vi "Effective degrees of freedom calculation.vi"(2 "nearest theoretical function from database":dbl[](array[numeric])=[14.666715524342548, 16.90138333280829, 19.565493531663716, 22.468034934420814, 25.369716242622864, 28.014507831534246, 30.16544604921263, 31.639384286174614, 32.33528562740709, 32.25150595291599, 31.48905866982018, 30.23994882008881, 28.76193292452598, 27.343183265376055, 26.26192732565865, 25.746976250071143, 25.94498751581365, 26.899339106940467, 28.543777449264834, 30.71179427774414, 33.160342822507424, 35.604375862397056, 37.75710565967028, 39.370078845854245, 40.26727255385307, 40.36834933783813, 39.69791434607072, 38.37971280154763, 36.61694734948651, 34.66188606250729, 32.77943678304789, 31.21009673576402, 30.137626105997057, 29.6659305163221, 29.80814246726195, 30.489001985309248, 31.55966117680997, 32.82225246541991, 34.06025124495686, 35.06998833065375, 35.68870706219568, 35.815289303031484, 35.42102179832661, 34.54938101853873, 33.30546999892364, 31.837235932372117, 30.311680207906562, 28.889849888622834, 27.704345150070246, 26.842494505993646, 26.337314169172064, 26.167078517448665, 26.262984518631317, 26.523216347810852, 26.830852818485937, 27.072649421221186, 27.155787017237554, 27.020182704278092, 26.644800169957563, 26.04742576452019, 25.27842670219093, 24.409909366263943, 23.522324470978415, 22.690824225874472, 21.973576014511963, 21.403769372456498, 20.986356362346143, 20.699733963447184, 20.50176337963178, 20.338847274488895, 20.156361380280483, 19.908603511423408, 19.566601960763993, 19.122562706598988, 18.5903545705075, 18.00211700795403, 17.40172856792016, 16.83636790594361, 16.347681467955717, 15.964091882344754, 15.695543683815888, 15.531549770559517, 15.442824584109177, 15.386191016951754, 15.311907534335774, 15.172173376651623, 14.929388720572566, 14.562800506093073, 14.072436542779842, 13.47967627959755, 12.82435029809701, 12.158818108287884, 11.539947216562274, 11.020255779363987, 10.639601442195865, 10.418718125431207, 10.355613818743219, 10.425399796133545, 10.583598834475756, 10.772447084026897, 10.929253846443201, 10.9955742344181, 10.925830234343435, 10.694101268139292, 10.298079096445033, 9.759604508936409, 9.121706289664775, 8.442574341744107, 7.787344576171037, 7.218879184426598, 6.788873197068151, 6.53055220457113, 6.453994560675933, 6.544726552242801, 6.765768046685836, 7.062816611730049, 7.37181710788848, 7.62783740408099, 7.77399991658564, 7.769226086789243, 7.593733645058184, 7.251551364867035, 6.7697423925322635, 6.1944854547659425, 5.584594642653517, 5.003403231784681, 4.510140742711135, 4.151991155059185, 3.9578971201764626, 3.93492274116682, 4.0676222706034215, 4.320445857712015, 4.642801727641996, 4.976042598414347, 5.261400575989181, 5.447787979996777, 5.49842305602821, 5.395421935934755, 5.141787446877443, 4.760589240715271, 4.291507174199621, 3.7852569778639444, 3.296687054103397, 2.8774871087765383, 2.569483917826434, 2.3993892663422827, 2.3756550396437954, 2.487793863704487, 2.708190092506199, 2.996098559817216, 3.303249852045647, 3.5802876217834663, 3.783176863206189, 3.878750413061122, 3.8486992279565726, 3.691532066743435, 3.4223110738347264, 3.070261929100643, 2.6746297226566798, 2.2793679210498117], 3 "experimental function":dbl[](array[numeric])=[22.30149557922684, 24.362732109266034, 27.297807376924123, 28.64644784708893, 30.248204511171004, 33.42077097860815, 34.59861401132268, 34.49590803669435, 34.45740788681342, 33.36138072141928, 33.135358407177556, 30.744170387682413, 31.818831427985444, 31.70369415417956, 31.13789549676162, 30.410402938882626, 30.775727742682065, 31.78984571089391, 31.856257108410997, 32.88897866912766, 31.82178580980581, 32.83420528522897, 33.46776374612122, 34.995645227686886, 34.254320967898096, 35.16210631396439, 34.582748836396554, 33.05477293030354, 32.107138663936055, 30.508586238189885, 28.742028842504045, 28.158263200159926, 27.730613373658617, 27.012013000747356, 26.76272642858672, 27.76579503861242, 29.12952017329807, 30.50064773668652, 32.347533632332905, 33.66314575155643, 34.485845630641116, 36.13419599571953, 37.803727241090854, 38.37709300881931, 37.848492410338146, 36.453703555710966, 34.51182843611985, 32.14306663838507, 29.481774615722255, 27.246665685952053, 26.08517191590534, 25.5801341551088, 25.19363770778496, 24.904957183804818, 24.758664278251384, 24.627305296072517, 24.38200827390981, 24.141227073887976, 24.084415331241505, 24.121016401846724, 24.003929701273606, 23.636991128095424, 23.106637504688006, 22.518409998010846, 21.995027001332055, 21.655930473064206, 21.501342518393606, 21.45593623464533, 21.423596336576153, 21.270528360159638, 20.866590470743613, 20.290821450884525, 19.786210205509146, 19.54819440948507, 19.49502981024729, 19.459861657507822, 19.31615977990748, 19.03410986955163, 18.597239600053566, 18.066972739018034, 17.604060080783324, 17.372003116353476, 17.34912949882708, 17.337388846583185, 17.137060625725994, 16.719937107229978, 16.200111296447833, 15.692335026769385, 15.201537947624546, 14.639731488586945, 13.916984884028617, 13.025964882566136, 12.042953978275785, 11.049929403040133, 10.13075635010201, 9.371052192583292, 8.857843057396456, 8.639406579154702, 8.676518923815488, 8.917180172662038, 9.301309755020757, 9.739719106382822, 10.134546476108095, 10.39659246387947, 10.526017588369776, 10.570457994989347, 10.57744273091549, 10.559856871290021, 10.492294201272376, 10.347170495184665, 10.120425909234006, 9.866225186214347, 9.648062536682414, 9.523799558676501, 9.51277775776358, 9.619255425023772, 9.844951843627971, 10.142138016542361, 10.416106848733088, 10.570010069752708, 10.542991249933042, 10.357363064046618, 10.04729070678893, 9.648839840648796, 9.20901112247331, 8.778973228709608, 8.406478566187976, 8.06986579533801, 7.683765220279402, 7.1609395986092235, 6.491627360905816, 5.830633566749115, 5.353591756383518, 5.188786374364739, 5.22176879240908, 5.2603191256959025, 5.126311620421436, 4.822570626106766, 4.480068818003462, 4.2301369000152675, 4.119333815319918, 4.074582090494102, 4.014110165818177, 3.8865877560275894, 3.7235372004501883, 3.5703759002554576, 3.4647319180085474, 3.4051304051891633, 3.3773819400179796, 3.3702433412070154, 3.399280743643882, 3.494776471163736, 3.6827044001330047, 3.9180423629733045, 4.096839785415113, 4.116858454500893, 3.9553122853005975, 3.681277972366111, 3.3679799057269713, 3.0665065289306415]) -> (0 "autocorrelation function":dbl[](graph)=[1.0, 0.9433836140832357, 0.8536129072370763, 0.7326741505053311, 0.6061175355222144, 0.4795219176188785, 0.3559784882733325, 0.2518198686036992, 0.17133591956659946, 0.11661480514181811, 0.08332996861979135, 0.06032561818746625, 0.051305730340803775, 0.03096129320892586, -0.003477211928289786, -0.04494342710752122, -0.09167249648218714, -0.1479822023477823, -0.20994698601085626, -0.26202934421660834, -0.30417307800211246, -0.31664588387655873, -0.30772271192602846, -0.2737317741240782, -0.22956081422876204, -0.1662065211480617, -0.10357026553691967, -0.04303830953070917, 0.01605018997696385, 0.06439122378368863, 0.0999002286031397, 0.12333212129030925, 0.13196224121500225, 0.13111001412755624, 0.12828750222158283, 0.12853575430052946, 0.13119472874222307, 0.13569574306640533, 0.14234330970095796, 0.14868838294289136, 0.15661402108672312, 0.1653330661989559, 0.1642195717693443, 0.1481407853631809, 0.12018965629953958, 0.08324645419853123, 0.0389434995118668, -0.010090478571855679, -0.05881599780861763, -0.1020011094385101, -0.13851507832731144, -0.1708377978525045, -0.1982498959131415, -0.2169075811596156, -0.2236912753895689, -0.21713398703146664, -0.19691498741518393, -0.16423216037318306, -0.1225970302911126, -0.07729331877408212, -0.03323712622387706, 0.006549547748027754, 0.040748606262771415, 0.0688748994157751, 0.09059757116228939, 0.10561780011777598, 0.11400220575334025, 0.11692319225892009, 0.11639493349975964, 0.11470427673290778, 0.11419707090007696, 0.11708899797187532, 0.12392689766414343, 0.13269503111991335, 0.13937782454869574, 0.14019449572107126, 0.1327937817876202, 0.11678770287752446, 0.09355693119362225, 0.06580278983787968, 0.036184833987804935, 0.0060561565839484565, -0.024636356017444412, -0.05599739175184271, -0.08693991558974715, -0.11511204955459801, -0.1381310885520937, -0.15482802332535708, -0.16563154822106263, -0.1718754705374281, -0.17478059279722416, -0.17505368657109616, -0.17291231241277932, -0.16835685581746304, -0.16097581812710368, -0.1502831283103745, -0.1360905904416939, -0.11861933729381714, -0.09820090130529095, -0.07485838966296518, -0.048597702630420306, -0.01966997798530354, 0.011399762117139091, 0.04385149336197631, 0.07696477628972742, 0.10994684439360028, 0.14173251761054087, 0.17077312404139336, 0.19522924099381533, 0.21341261644600892, 0.22417507623554067, 0.22680800927242878, 0.221266050917819, 0.20883185429880127, 0.1919551759778061, 0.17308740307722767, 0.1542668283802011, 0.1369836344131975, 0.1226675783538473, 0.11283491146887599, 0.10780212361189712, 0.10653939909485778, 0.10772091760541626, 0.10979629459063298, 0.11069442055141408, 0.10927149498494101, 0.1043917754185449, 0.0944056997119095, 0.07884071707582518, 0.05917125383383133, 0.03818214486838395, 0.01870039400781659, 0.0036102196648571177, -0.005543712195955346, -0.009923374258118537, -0.00998005745328413, -0.005414614826691831, 0.0022717653890917287, 0.01397453123294509, 0.027281772765425625, 0.0398135874061571, 0.04739543770789759, 0.050130408820784185, 0.04753757233188854, 0.04176724136497284, 0.0341874291801756, 0.025668409659487957, 0.01764628589160147, 0.011529704885510804, 0.009048268747577165, 0.008134312150999847, 0.010035757122124598, 0.013065780403137384, 0.016186260327724234, 0.017595748729977077, 0.017143241991131077, 0.016101474410560448, 0.01360068215802751, 0.009537045850078215, 0.005132596032725284], 1 "effective degrees of freedom":dbl=16.453036115287905)   [LabVIEW 2018]
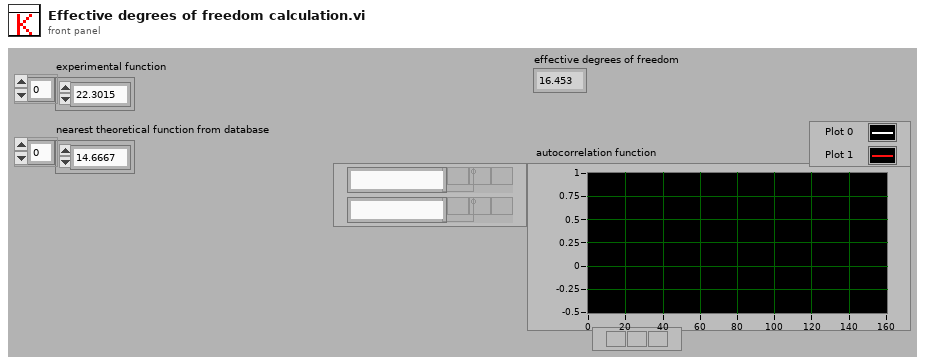
[diagram p1: front panel]
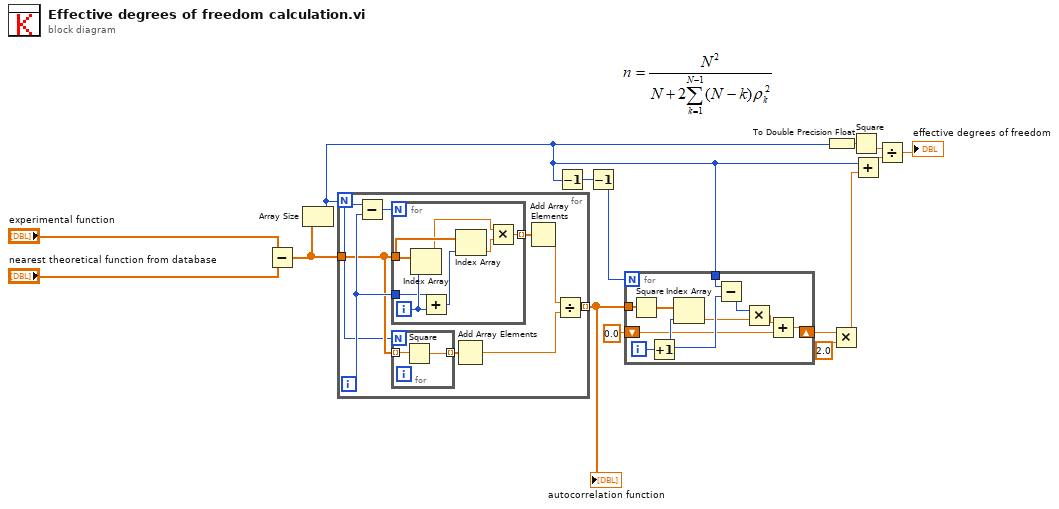
[diagram p0: block diagram]
diagram:
  n1 = Subtract(x="experimental function", y="nearest theoretical function from database") -> (x-y=w5:dbl[])
  n2 = Array Size(array=w5) -> (size(s)=w8:i32)
  n3 = for {
    N: w8 -> [w16]
    tunnel: w5 -> [w21]
    tunnel: [w18] -> w2 mode=indexing
    i -> [w24]
    n4 = Subtract(x=w16, y=w24) -> (x-y=w17:i32)
    n5 = for {
      N: w17 -> [_]
      tunnel: w21 -> [w33]
      tunnel: [w29] -> w23 mode=indexing
      tunnel: w24 -> [w27]
      i -> [w32]
      n6 = Index Array(array=w33, index=w32) -> (element=w30:dbl)
      n7 = Add(x=w27, y=w32) -> (x+y=w28:i32)
      n8 = Index Array(array=w33, index=w28) -> (element=w31:dbl)
      n9 = Multiply(x=w30, y=w31) -> (x*y=w29:dbl)
    }
    n10 = for {
      N: w16 -> [_]
      tunnel: w21 -> [w26] mode=indexing
      tunnel: [w25] -> w22 mode=indexing
      n11 = Square(x=w26) -> (x^2=w25:dbl)
    }
    n12 = Add Array Elements(numeric array=w22) -> (sum=w19:dbl)
    n13 = Add Array Elements(numeric array=w23) -> (sum=w20:dbl)
    n14 = Divide(x=w20, y=w19) -> (x/y=w18:dbl)
  }
  "autocorrelation function" <- w2
  n15 = Decrement(x=w8) -> (x-1=w9:i32)
  n16 = Decrement(x=w9) -> (x-1=w10:i32)
  n17 = for {
    N: w10 -> [_]
    tunnel: w2 -> [w37]
    tunnel: w8 -> [w42]
    shift-right: [w34] -> w3
    shift-left: 0.0 -> [w35]
    i -> [w43]
    n18 = Square(x=w37) -> (x^2=w38:dbl[])
    n19 = Increment(x=w43) -> (x+1=w41:i32)
    n20 = Index Array(array=w38, index=w41) -> (element=w39:dbl)
    n21 = Subtract(x=w42, y=w41) -> (x-y=w40:i32)
    n22 = Multiply(x=w40, y=w39) -> (x*y=w36:dbl)
    n23 = Add(x=w36, y=w35) -> (x+y=w34:dbl)
  }
  n24 = To Double Precision Float(number=w8) -> (double precision float=w1:dbl)
  n25 = Multiply(x=w3, y=2.0 ("x")) -> (x*y=w14:dbl)
  n26 = Square(x=w1) -> (x^2=w12:dbl)
  n27 = Add(x=w8, y=w14) -> (x+y=w13:dbl)
  n28 = Divide(x=w12, y=w13) -> (x/y=→"effective degrees of freedom":dbl)
